vi "Replace Board Pixel.vi"(8 "error in (no error)":errorcluster, 9 "Colour":u32(colorbox), 10 "Coordinates":T1, 11 "Game Board in":refnum<class "Game Board.lvclass">) -> (0 "error out":errorcluster, 3 "Game Board out":refnum<class "Game Board.lvclass">)   [LabVIEW 2018, in "Game Board.lvclass"]
uses:
  Game Board.lvclass
  Snake/Type Defs/Coordinates.ctl
  Game Board.lvclass/Game Board.ctl
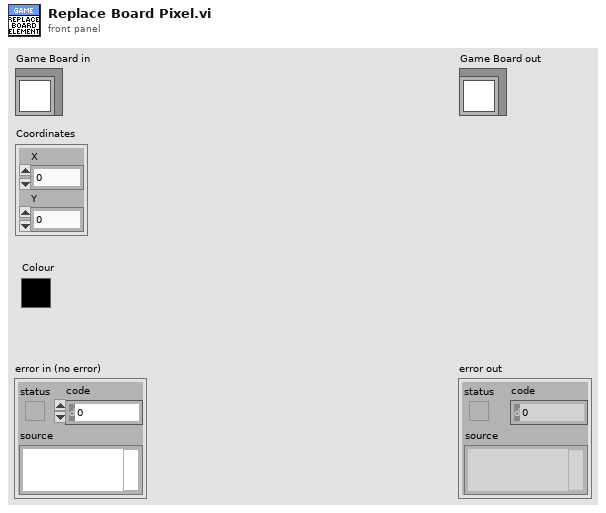
[diagram p1: front panel]
types:
  T1 = typedef "Coordinates.ctl" = cluster{"X":i32, "Y":i32}
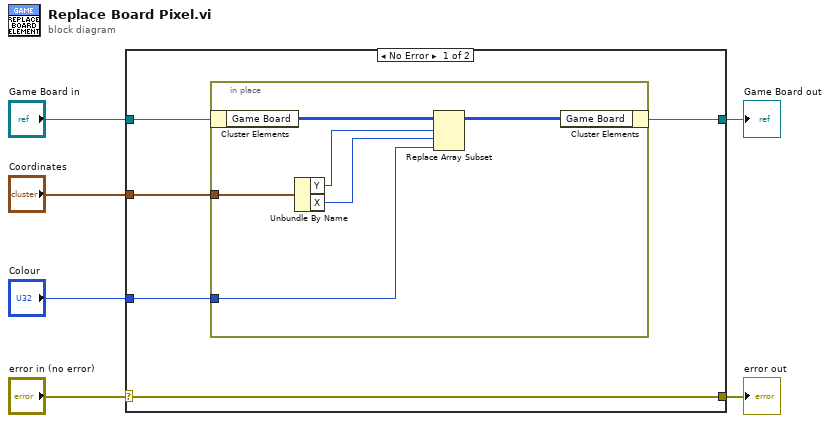
[diagram p0: block diagram]
diagram:
  n1 = case shown="No Error" "error in (no error)" {
    selector: "error in (no error)" -> [w11 w19]
    tunnel: [w11 w19] -> w5
    tunnel: [w7 w18] -> w3
    tunnel: "Game Board in" -> [w10 w18]
    tunnel: "Colour" -> [w9 _]
    tunnel: "Coordinates" -> [w8 _]
    frame No Error {
      n2 = in-place {
        in-place-border: w9 -> [w15]
        in-place-border: w8 -> [w14]
        n3 = in-place-cluster #1(w10) -> ("Game Board"=w17:u32[][])
        n4 = Unbundle By Name(w14) -> ("Y"=w13:i32, "X"=w12:i32)
        n5 = Replace Array Subset(array=w17, new element=w15, index (row)=w13, index (col)=w12) -> (w16:u32[][])
        n6 = in-place-cluster #1("Game Board"=w16) -> (w7:refnum<class "Game Board.lvclass">)
      }
    }
    frame Error {
    }
  }
  "error out" <- w5
  "Game Board out" <- w3
